vi "AmpelBR.vi"() -> ()   [LabVIEW 2024]
uses:
  <vilib>/OPCUA/controls/NodeIds.ctl
  <vilib>/OPCUA/controls/NodeId.ctl
  <vilib>/OPCUA/client/Multiple Read Bool.vi
  <vilib>/OPCUA/client/Multiple Read Byte.vi
  <vilib>/OPCUA/NI OPC UA Client.lvlib
panel:
  out "CountDown":u8
  out "Green":bool
  out "Yellow":bool
  out "Red":bool
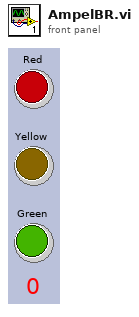
[diagram p1: front panel]
types:
  T1 = typedef "NodeIds.ctl" = T2[]
  T2 = typedef "NodeId.ctl" = string
  T3 = typedef "OPC UA Client Refnum.ctl" = refnum<k21>
  T4 = typedef "OPC UA StatusCode.ctl" = u32
  T5 = cluster{"node ID":T2, "value ":u8, "timestamp":timestamp, "status":T4}[]
  T6 = cluster{"node ID":T2, "value ":bool, "timestamp":timestamp, "status":T4}[]
  T7 = cluster{"node ID":T2, "value ":u8, "timestamp":timestamp, "status":T4}
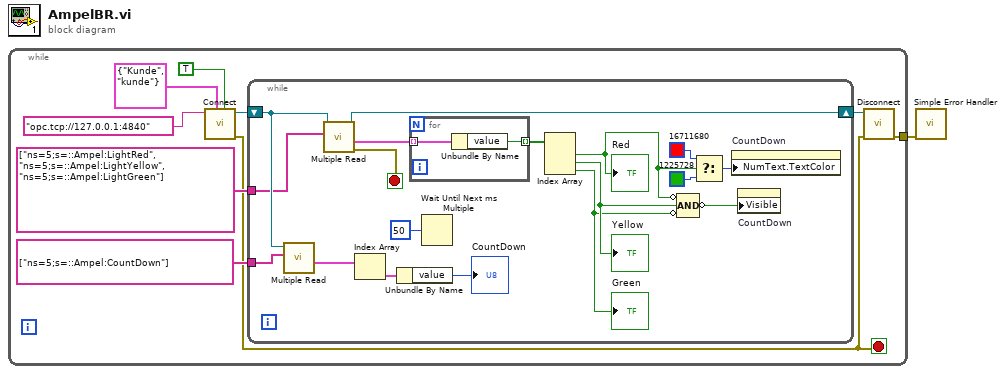
[diagram p0: block diagram]
diagram:
  n1 = while {
    tunnel: [w8] -> w1
    stop <- w2 stop-if-true
    n2 = call <vilib>:"Connect.vi"("trust any server (F)"=TRUE, "username/password"=cluster{"username":string, "password":string} {"username"="Kunde", "password"="kunde"}, "server endpoint URL"="opc.tcp://127.0.0.1:4840") -> ("error out"=w2:errorcluster, "OPC UA client refnum out"=w6:T3)  [unwired: 6 in, 1 out]
    n3 = while {
      shift-right: [w27] -> w5
      shift-left: w6 -> [w24]
      tunnel: T1 ["ns=5;s=::Ampel:CountDown"] ("node IDs") -> [w15]
      tunnel: T1 ["ns=5;s=::Ampel:LightRed", "ns=5;s=::Ampel:LightYellow", "ns=5;s=::Ampel:LightGreen"] ("node IDs") -> [w14]
      stop <- w13 stop-if-true
      n4 = call-poly <vilib>:"Multiple Read.vi"("node IDs"=w15, "OPC UA client refnum in"=w24) -> ("results"=w23:T5)  [unwired: 6 in, 3 out]
      n5 = call-poly <vilib>:"Multiple Read.vi"("node IDs"=w14, "OPC UA client refnum in"=w24) -> ("error out"=w13:errorcluster, "results"=w28:T6, "OPC UA client refnum out"=w27:T3)  [unwired: 6 in, 1 out]
      n6 = Index Array(array=w23) -> (element=w22:T7)  [unwired: 1 in]
      n7 = Unbundle By Name(w22) -> ("value"=→"CountDown":u8)
      n8 = for {
        tunnel: w28 -> [w30] mode=indexing
        tunnel: [w29] -> w25 mode=indexing
        n9 = Unbundle By Name(w30) -> ("value"=w29:bool)
      }
      n10 = Wait Until Next ms Multiple(millisecond multiple=u32 50) -> ()  [unwired: 1 out]
      n11 = Index Array(array=w25) -> (element #1=w11:bool, element #2=w17:bool, element #3=w12:bool)  [unwired: 3 in]
      "Red" <- w11
      "Yellow" <- w17
      "Green" <- w12
      n12 = Compound Arithmetic op=AND(invert w11, w17, invert w12) -> (invert w16:bool)
      n13 = Select(t=u32 16711680, s=w11, f=u32 1225728) -> (s? t:f=w18:u32)
      n14 = property on="CountDown" class="DigNum (strict)"("NumText.TextColor"=w18) -> ()  [unwired: 2 in, 2 out]
      n15 = property on="CountDown" class="DigNum (strict)"("Visible"=w16) -> ()  [unwired: 2 in, 2 out]
    }
    n16 = call <vilib>:"Disconnect.vi"("error in (no error)"=w2, "OPC UA client refnum in"=w5) -> ("error out"=w8:errorcluster)  [unwired: 9 in]
  }
  n17 = call <vilib>:"Simple Error Handler.vi"("error in (no error)"=w1) -> ()  [unwired: 4 in, 5 out]
